vi "DataLog Strip Meta Specifier.vi"(7 "tag":string) -> (4 "meta specifier":T1, 8 "base tag":string)   [LabVIEW 2012]
doc: "Takes a tag and tries to remove the meta specifier from its ending. The base tag and meta specifier enum are returned. When the tag does not correspond to a meta channel, \"not a meta\" and the original tag are returned. This VI is the inverse of \"Append Meta Specifier\"."
uses:
  typedefs/et_DataLog Meta Tag Specifier.ctl
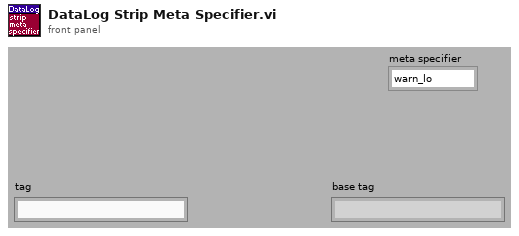
[diagram p1: front panel]
types:
  T1 = typedef "et_DataLog Meta Tag Specifier.ctl" = enum32{"warn_lo", "warn_hi", "A_lo", "A_hi", "B_lo", "B_hi", "C_lo", "C_hi", "D_lo", "D_hi", "E_lo", "E_hi", "F_lo", "F_hi", "G_lo", "G_hi", "H_lo", "H_hi", "I_lo", "I_hi", "J_lo", "J_hi", "K_lo", "K_hi", "L_lo", "L_hi", "M_lo", "M_hi", "N_lo", "N_hi", "min", "max", "not a meta"}
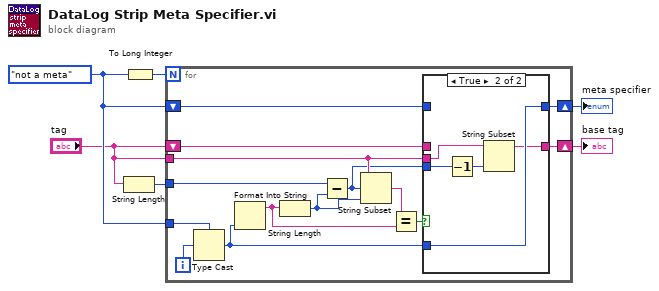
[diagram p0: block diagram]
diagram:
  w4 = et_DataLog_Meta_Tag_Specifier."not a meta" ("meta specifier (not a meta)")
  n1 = String Length(string="tag") -> (length=w1:i32)
  n2 = To Long Integer(number=w4) -> (32bit integer=w6:i32)
  n3 = for {
    N: w6 -> [_]
    shift-right: [w14] -> w5
    shift-left: w4 -> [w13]
    shift-right: [w11] -> w3
    shift-left: "tag" -> [w12]
    tunnel: w4 -> [w20]
    tunnel: "tag" -> [w9]
    tunnel: w1 -> [w8]
    i -> [w19]
    n4 = Type Cast(type=w20, x=w19) -> (*(type *) &x=w10:T1)
    n5 = Format Into String(w10) -> (resulting string=w16:string)  [unwired: 3 in, 1 out]
    n6 = String Length(string=w16) -> (length=w18:i32)
    n7 = Subtract(x=w8, y=w18) -> (x-y=w7:i32)
    n8 = String Subset(string=w9, offset (0)=w7, length (rest)=w18) -> (substring=w17:string)
    n9 = Equal?(x=w17, y=w16) -> (x = y?=w15:bool)
    n10 = case shown="True" w15 {
      tunnel: w13 -> [w22 _]
      tunnel: [w22 w27] -> w14
      tunnel: w12 -> [w21 _]
      tunnel: [w21 w23] -> w11
      tunnel: w10 -> [_ w27]
      tunnel: w7 -> [_ w26]
      tunnel: w9 -> [_ w24]
      frame False {
      }
      frame True {
        n11 = Decrement(x=w26) -> (x-1=w25:i32)
        n12 = String Subset(string=w24, length (rest)=w25) -> (substring=w23:string)  [unwired: 1 in]
      }
    }
  }
  "meta specifier" <- w5
  "base tag" <- w3
